vi "filter_to_zero_pole_gain.vi"(6 "Fs":dbl, 10 "IIR Filter Cluster":T2 {"Forward Coefficients" format="%#_4g"; "Reverse Coefficients" format="%#_4g"}) -> (2 "Zero/Pole/Gain":cluster{" Zeros":T1[], "Poles":T1[], "Gain":dbl}={" Zeros"=[], "Poles"=[], "Gain"=1.0} {"Poles"."Frequency" format="%#_3p"; "Poles"."Damping" min=0.0 max=1000.0 step=1.0 format="%#_3g"; "Zeros"."Frequency" format="%#_3p"; "Zeros"."Damping" min=0.0 max=1000.0 step=1.0 format="%#_3g"})   [LabVIEW 2010]
uses:
  damping_freq.ctl
panel:
  # "Convert a Labview IIR cascade filter into pole/zero/gain representation, where the poles and zeros are represented by frequency and damping and the gain is the DC gain.  Inverse of zero_pole_gain_to_filter"
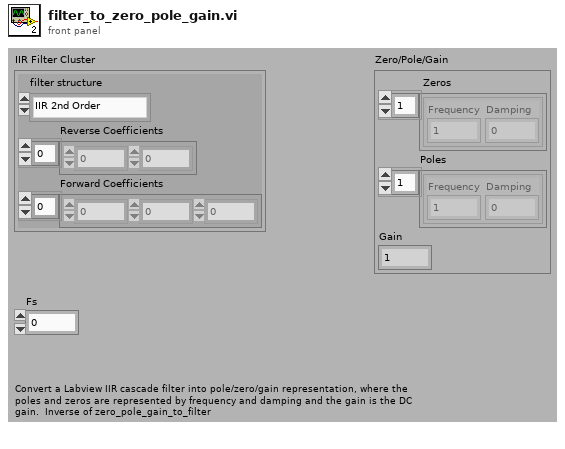
[diagram p1: front panel]
types:
  T1 = typedef "damping_freq.ctl" = cluster{"Frequency":dbl, "Damping":dbl}
  T2 = cluster{"filter structure":enum32{"IIR 2nd Order", "IIR 4th Order"}, "Reverse Coefficients":dbl[], "Forward Coefficients":dbl[]}
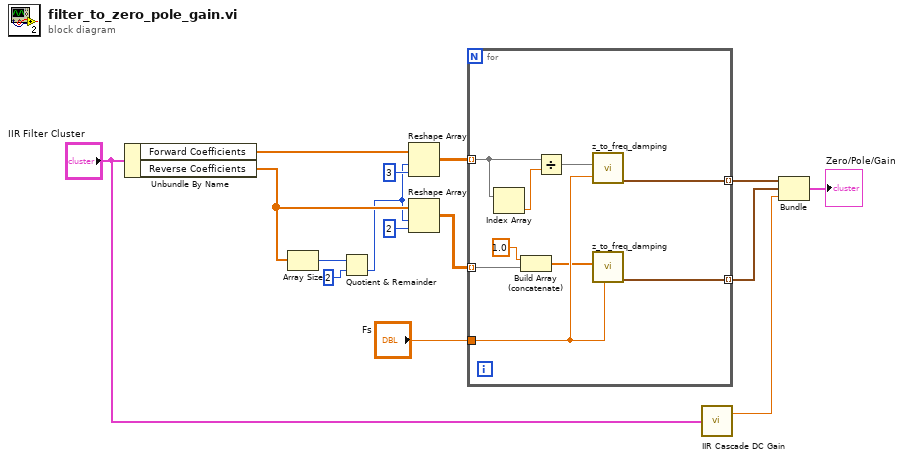
[diagram p0: block diagram]
diagram:
  n1 = Unbundle By Name("IIR Filter Cluster") -> ("Forward Coefficients"=w9:dbl[], "Reverse Coefficients"=w10:dbl[])
  n2 = Array Size(array=w10) -> (size(s)=w14:i32)
  n3 = Quotient & Remainder(x=w14, y=2) -> (floor(x/y)=w6:i32)  [unwired: 1 out]
  n4 = Reshape Array(w9, w6, 3 ("dimension size")) -> (w7:dbl[][])
  n5 = Reshape Array(w10, w6, 2 ("dimension size")) -> (w8:dbl[][])
  n6 = for {
    tunnel: w8 -> [w23] mode=indexing
    tunnel: w7 -> [w18] mode=indexing
    tunnel: "Fs" -> [w24]
    tunnel: [w20] -> w4 mode=indexing
    tunnel: [w19] -> w5 mode=indexing
    n7 = Index Array(array=w18) -> (element=w17:dbl)  [unwired: 1 in]
    n8 = Build Array (concatenate)(1.0 ("Fs"), w23) -> (w21:dbl[])
    n9 = Divide(x=w18, y=w17) -> (x/y=w16:dbl[])
    n10 = call "z_to_freq_damping.vi"("Fs"=w24, "Coefficients"=w16) -> ("Characteristics"=w19:T1)  [unwired: 9 out]
    n11 = call "z_to_freq_damping.vi"("Fs"=w24, "Coefficients"=w21) -> ("Characteristics"=w20:T1)  [unwired: 9 out]
  }
  n12 = call "IIR Cascade DC Gain.vi"("IIR Filter Cluster"="IIR Filter Cluster") -> ("Gain"=w1:dbl)  [unwired: 4 out]
  n13 = Bundle(w5, w4, "Gain"=w1) -> (→"Zero/Pole/Gain":cluster{T1[], T1[], "Gain":dbl})  [unwired: 1 out]
